vi "Make Configuration Array.vi"(8 "Error In":errorcluster, 9 "Number of components":i32, 10 "Index Array":i32[][](array[numeric]), 11 "Tab Page Ref":refnum<vi>[](array[refnum])) -> (0 "Error Out":errorcluster, 1 "no. Updates":u32, 2 "New Configuration":string[](array[string]), 3 "Tab Page Ref dup":refnum<vi>[](array[refnum]))   [LabVIEW 2014]
doc: "This VI finds updates. It builds an array for new configuration according to the TDMS file order. It also updates the boolean array according to updates. \n\nIf the new version field is empty or equal to the current version field, it copies the current version field. \nIf the new version field is updated, it copies the new version field, and reconizes this as an update."
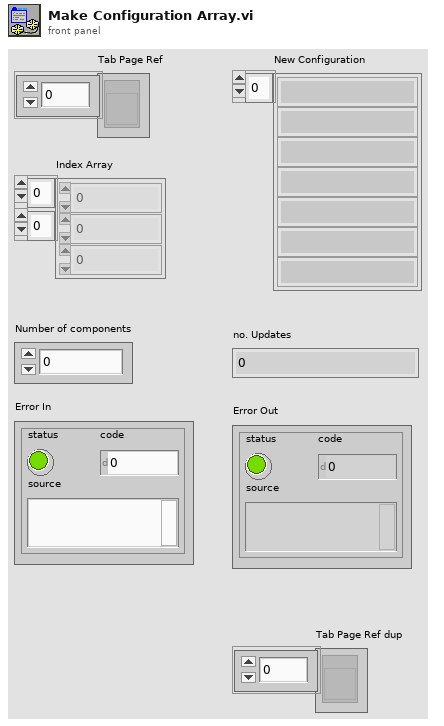
[diagram p1: front panel]
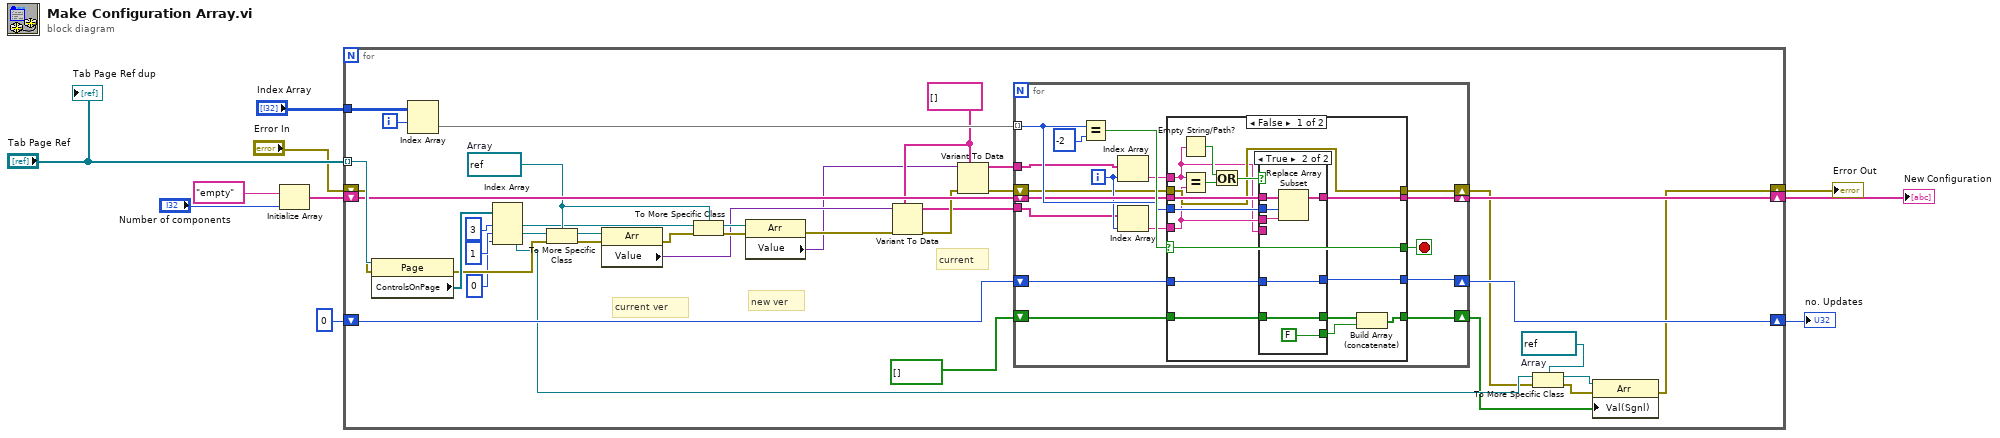
[diagram p0: block diagram]
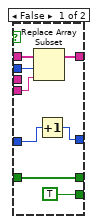
[diagram p2: hidden frame]
diagram:
  n1 = Initialize Array("empty", "Number of components") -> (w4:string[])
  n2 = for {
    tunnel: "Tab Page Ref" -> [w48] mode=indexing
    shift-right: [w11] -> w8
    shift-left: "Error In" -> [w47]
    tunnel: "Index Array" -> [w39]
    shift-right: [w40] -> w6
    shift-left: w4 -> [w44]
    shift-right: [w20] -> w1
    shift-left: u32 0 ("Dial") -> [w21]
    i -> [w37]
    w17 = refnum<vi> refnum  # Array
    w28 = string[] []
    w35 = refnum<vi> refnum  # Array
    # "current"
    # "new ver"
    # "current ver"
    n3 = property class="Page"(reference=w48, error in=w47) -> (error out=w36:errorcluster, "ControlsOnPage"=w46:refnum<vi>[])  [unwired: 1 out]
    n4 = Index Array(array=w39, index (row)=w37) -> (element=w38:i32[])  [unwired: 1 in]
    n5 = Index Array(array=w46, index #1=3 ("index"), index #2=1 ("index"), index #3=0 ("index")) -> (element #1=w34:refnum<vi>, element #2=w42:refnum<vi>, element #3=w14:refnum<vi>)
    n6 = To More Specific Class(target class=w35, reference=w42, error in=w36) -> (specific class reference=w32:refnum<vi>, error out=w33:errorcluster)
    n7 = property class="Arr"(reference=w32, error in=w33) -> (error out=w31:errorcluster, "Value"=w25:variant)  [unwired: 1 out]
    n8 = To More Specific Class(target class=w35, reference=w34, error in=w31) -> (specific class reference=w29:refnum<vi>, error out=w30:errorcluster)
    n9 = property class="Arr"(reference=w29, error in=w30) -> (error out=w26:errorcluster, "Value"=w24:variant)  [unwired: 1 out]
    n10 = Variant To Data(error in=w26, type=w28, Variant=w25) -> (data=w23:string[], error out=w27:errorcluster)
    n11 = Variant To Data(error in=w27, type=w28, Variant=w24) -> (data=w41:string[], error out=w22:errorcluster)
    n12 = for {
      tunnel: w38 -> [w62] mode=indexing
      tunnel: w41 -> [w54]
      shift-right: [w60] -> w40
      shift-left: w44 -> [w61]
      tunnel: w23 -> [w53]
      shift-right: [w55] -> w12
      shift-left: w22 -> [w56]
      shift-right: [w51] -> w20
      shift-left: w21 -> [w52]
      shift-right: [w50] -> w13
      shift-left: bool[] [] -> [w49]
      i -> [w58]
      stop <- w63 stop-if-true
      n13 = Equal?(x=w62, y=-2) -> (x = y?=w64:bool)
      n14 = Index Array(array=w54, index=w58) -> (element=w59:string)
      n15 = Index Array(array=w53, index=w58) -> (element=w57:string)
      n16 = case shown="False" w64 {
        selector: w64 -> [w75 w101]
        tunnel: [w75 w101] -> w63
        tunnel: w62 -> [w77 _]
        tunnel: w61 -> [w78 w100]
        tunnel: w59 -> [w72 _]
        tunnel: w57 -> [w73 _]
        tunnel: [w76 w100] -> w60
        tunnel: w56 -> [w74 w99]
        tunnel: [w74 w99] -> w55
        tunnel: w52 -> [w71 w98]
        tunnel: [w70 w98] -> w51
        tunnel: [w69 w97] -> w50
        tunnel: w49 -> [w67 w97]
        frame False {
          n17 = Empty String/Path?(string/path=w72) -> (empty?=w80:bool)
          n18 = Equal?(x=w72, y=w73) -> (x = y?=w81:bool)
          n19 = Or(x=w80, y=w81) -> (x .or. y?=w79:bool)
          n20 = case shown="True" w79 {
            tunnel: w78 -> [w89 w96]
            tunnel: w77 -> [w88 w95]
            tunnel: w73 -> [_ w93]
            tunnel: [w87 w94] -> w76
            tunnel: w72 -> [w86 _]
            tunnel: w71 -> [w85 w92]
            tunnel: [w84 w92] -> w70
            tunnel: [w83 w91] -> w68
            tunnel: w67 -> [w83 w91]
            tunnel: [TRUE FALSE] -> w66
            frame False {
              n21 = Replace Array Subset(array=w89, new element=w86, index=w88) -> (w87:string[])
              n22 = Increment(x=w85) -> (x+1=w84:u32)
            }
            frame True {
              n23 = Replace Array Subset(array=w96, new element=w93, index=w95) -> (w94:string[])
            }
          }
          n24 = Build Array (concatenate)(w68, w66) -> (w69:bool[])
        }
        frame True {
        }
      }
    }
    n25 = To More Specific Class(target class=w17, reference=w14, error in=w12) -> (specific class reference=w15:refnum<vi>, error out=w16:errorcluster)
    n26 = property class="Arr"(reference=w15, error in=w16, "Val(Sgnl)"=w13) -> (error out=w11:errorcluster)  [unwired: 1 out]
  }
  "Error Out" <- w8
  "New Configuration" <- w6
  "no. Updates" <- w1
  "Tab Page Ref dup" <- "Tab Page Ref"
